vi "PI_GCS3_Sample_Application_Motion.vi"() -> ()   [LabVIEW 2020]
doc: "This VI demonstrates how to initialize a PI GCS3 system and how to query the help answer. \nThe diagram shows how to combine the driver VIs for these tasks. \n\nWarning: Before running this VI, modify the interface settings on the block diagram to reflect your configuration. The predefined settings provided with the VI probably do not match your system.\n\nCompatibility: This sample requires a PI GCS 3.0 controller."
uses:
  Interface Settings.ctl
  ModeOfOperation.ctl
panel:
  out "All axes on target?":bool
  out "All axes referenced?":bool
  out "Axes available?":bool caption="Any axes available?"
  out "Axis on target?":bool[](array[boolean])
  out "Referenced?":bool[](array[boolean])
  out "Any axes moving?":bool
  in  "Target Position":dbl[](array[numeric]) format="%.6f"
  out "Current Position":dbl[](array[numeric]) format="%.6f"
  in  "stop":bool
  in  "error in":errorcluster
  out "Running":bool caption="Configuration_Setup.vi is running"
  out "error out":errorcluster
  out "Conn. Axis":string[](array[string])
  out "Identification":string
  # "This VI demonstrates how to initialize a PI GCS3 system and how to move your axes.\nThe diagram shows how to combine the driver VIs for these tasks. \n\nWarning: Before running this VI, modify the interface settings on the block diagram to reflect your configuration.\n                 The predefined settings provided with the VI probably do not match your system.\n\nCompatibility: This sample requires a PI GCS 3.0 controller."
  # "Set the number of target positions\naccording to your connected axes."
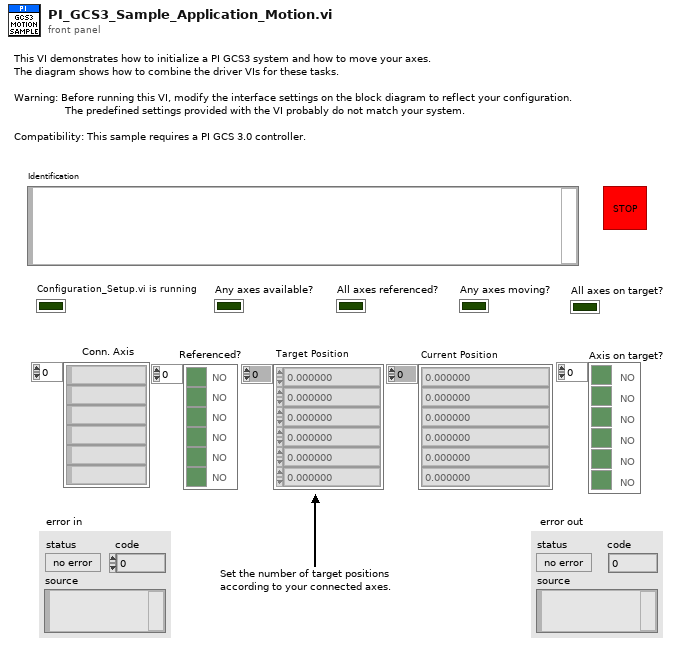
[diagram p1: front panel]
types:
  T1 = typedef "ModeOfOperation.ctl" = enum16{"Open", "Open-Loop Position", "Closed-Loop Position", "Open-Loop Velocity", "Closed-Loop Velocity", "Open-Loop Force", "Closed-Loop Force", "Step Operation"}
  T2 = typedef "Interface Settings.ctl" = cluster{"Interface":u16, "Timeout":u32, "RS232 settings":cluster{"Portnumber":u8, "Baudrate":u16}, "TCP/IP settings":cluster{"Host address/name":string, "Port":i32, "Board":i32, "TCP/IP Search?":bool}, "USB settings":cluster{"S/N":string, "USB Search?":bool}, "DaisyChain settings":cluster{"Register DC":bool, "DaisyChain Search?":bool, "Device ID":i32}, "DLL for Device":u16}
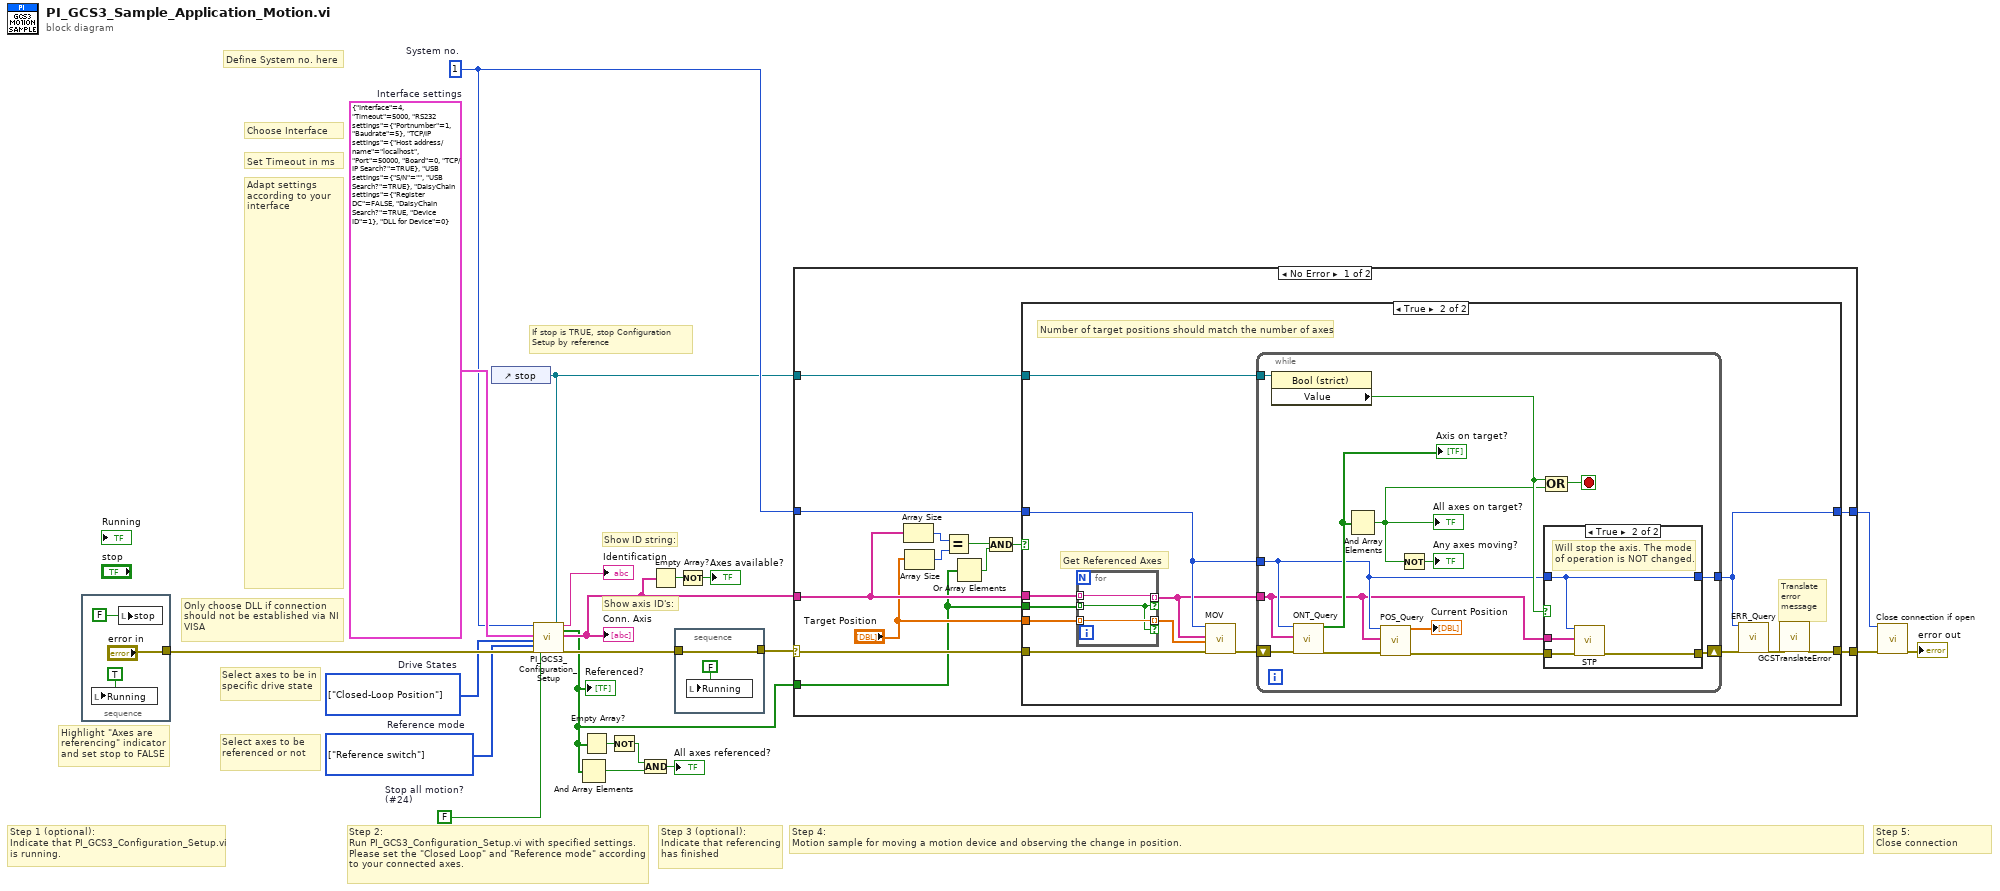
[diagram p0: block diagram]
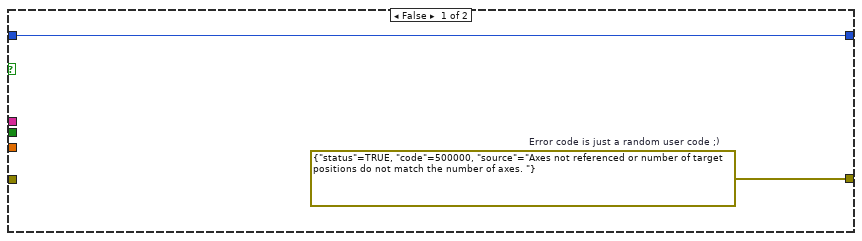
[diagram p2: hidden frame]
diagram:
  w1 = enum16{"Do not reference", "Reference switch"}[] [enum."Reference switch"] items=["Do not reference", "Reference switch"]  # Reference mode
  w2 = T1[] [enum."Closed-Loop Position"] items=["Open", "Open-Loop Position", "Closed-Loop Position", "Open-Loop Velocity", "Closed-Loop Velocity", "Open-Loop Force", "Closed-Loop Force", "Step Operation"]  # Drive States
  w16 = T2 {"Interface"=4, "Timeout"=5000, "RS232 settings"={"Portnumber"=1, "Baudrate"=5}, "TCP/IP settings"={"Host address/name"="localhost", "Port"=50000, "Board"=0, "TCP/IP Search?"=TRUE}, "USB settings"={"S/N"="", "USB Search?"=TRUE}, "DaisyChain settings"={"Register DC"=FALSE, "DaisyChain Search?"=TRUE, "Device ID"=1}, "DLL for Device"=0}  # Interface settings
  w17 = FALSE  # Stop all motion? (#24)
  w13 = 1  # System no.
  # "Step 5:\nClose connection"
  # "Define System no. here"
  # "Select axes to be referenced or not"
  # "Select axes to be in specific drive state"
  # "Adapt settings according to your interface"
  # "Set Timeout in ms"
  # "Choose Interface"
  # "Only choose DLL if connection should not be established via NI VISA"
  # "If stop is TRUE, stop Configuration\nSetup by reference"
  # "Step 4: \nMotion sample for moving a motion device and observing the change in position."
  # "Step 3 (optional): \nIndicate that referencing has finished"
  # "Step 2: \nRun PI_GCS3_Configuration_Setup.vi with specified settings.\nPlease set the \"Closed Loop\" and \"Reference mode\" according\nto your connected axes."
  # "Step 1 (optional): \nIndicate that PI_GCS3_Configuration_Setup.vi is running."
  # "Highlight \"Axes are\nreferencing\" indicator\nand set stop to FALSE"
  # "Show axis ID's:"
  # "Show ID string:"
  n1 = stacked-sequence {
    tunnel: ["error in"] -> w20
    frame #0 {
      n2 = local write "Running"(TRUE ("Running")) -> ()
      n3 = local write "stop"(FALSE ("stop")) -> ()
    }
  }
  n4 = control-ref of="stop"() -> (w12:refnum<vi>)
  n5 = call "PI_GCS3_Configuration_Setup.vi"("System no."=w13, "Interface settings"=w16, "Mode of operation"=w2, "Reference mode"=w1, "error in"=w20, "Stop all motion?"=w17, "Stop refnum"=w12) -> ("Identification"=→"Identification":string, "Referenced?"=w6:bool[], "Conn. axis"=w8:string[], "error out"=w19:errorcluster)  [unwired: 7 in, 2 out]
  "Conn. Axis" <- w8
  "Referenced?" <- w6
  n6 = And Array Elements(Boolean array=w6) -> (logical AND=w3:bool)
  n7 = Empty Array?(array=w6) -> (empty?=w7:bool)
  n8 = Not(x=w7) -> (.not. x?=w4:bool)
  n9 = And(x=w4, y=w3) -> (x .and. y?=→"All axes referenced?":bool)
  n10 = Empty Array?(array=w8) -> (empty?=w10:bool)
  n11 = stacked-sequence {
    tunnel: w19 -> [w25]
    tunnel: [w25] -> w15
    frame #0 {
      n12 = local write "Running"(FALSE ("Running")) -> ()
    }
  }
  n13 = Not(x=w10) -> (.not. x?=→"Axes available?":bool)
  n14 = case shown="No Error" w15 {
    selector: w15 -> [w28 w79]
    tunnel: [w39 w79] -> w11
    tunnel: w13 -> [w37 w78]
    tunnel: [w38 w78] -> w14
    tunnel: w8 -> [w35 _]
    tunnel: w12 -> [w36 _]
    tunnel: w6 -> [w27 _]
    frame No Error {
      n15 = Array Size(array=w35) -> (size(s)=w33:i32)
      n16 = Array Size(array="Target Position") -> (size(s)=w32:i32)
      n17 = Equal?(x=w33, y=w32) -> (x = y?=w31:bool)
      n18 = Or Array Elements(Boolean array=w27) -> (logical OR=w29:bool)
      n19 = And(x=w31, y=w29) -> (x .and. y?=w30:bool)
      n20 = case shown="True" w30 {
        tunnel: [w40 w54] -> w39
        tunnel: w28 -> [_ w52]
        tunnel: [w41 w50] -> w38
        tunnel: w35 -> [_ w49]
        tunnel: w27 -> [_ w48]
        tunnel: w37 -> [w41 w47]
        tunnel: w36 -> [_ w45]
        tunnel: "Target Position" -> [_ w43]
        frame False {
          w40 = errorcluster {"status"=TRUE, "code"=500000, "source"="Axes not referenced or number of target positions do not match the number of axes. "}  # Error code is just a random user code ;)
        }
        frame True {
          # "Number of target positions should match the number of axes"
          # "Get Referenced Axes"
          # "Translate\nerror \nmessage"
          n21 = for {
            tunnel: w49 -> [w57] mode=indexing
            tunnel: w48 -> [w55] mode=indexing
            tunnel: [w57] -> w46 mode=indexing if=w55
            tunnel: [w56] -> w42 mode=indexing if=w55
            tunnel: w43 -> [w56] mode=indexing
          }
          n22 = call "MOV.vi"("System no."=w47, "Axes to move"=w46, "Position values"=w42, "error in"=w52) -> ("error out"=w44:errorcluster)  [unwired: 1 in, 14 out]
          n23 = while {
            shift-right: [w69] -> w51
            shift-left: w44 -> [w63]
            tunnel: w45 -> [w68]
            tunnel: w47 -> [w62]
            tunnel: w46 -> [w61]
            tunnel: [w64] -> w50
            stop <- w67 stop-if-true
            n24 = property class="Bool (strict)"(reference=w68) -> ("Value"=w66:bool)  [unwired: 1 in, 2 out]
            n25 = call "ONT_Query.vi"("System no."=w62, "Axes to query"=w61, "error in"=w63) -> ("Axis on target?"=w65:bool[], "error out"=w71:errorcluster)  [unwired: 2 in, 13 out]
            "Axis on target?" <- w65
            n26 = And Array Elements(Boolean array=w65) -> (logical AND=w58:bool)
            "All axes on target?" <- w58
            n27 = call "POS_Query.vi"("System no."=w62, "Axes to query"=w61, "error in"=w71) -> ("Position"=→"Current Position":dbl[], "error out"=w70:errorcluster)  [unwired: 2 in, 13 out]
            n28 = Not(x=w58) -> (.not. x?=→"Any axes moving?":bool)
            n29 = case shown="True" w66 {
              tunnel: w70 -> [w73 w76]
              tunnel: [w73 w75] -> w69
              tunnel: w62 -> [w72 w77]
              tunnel: [w72 w77] -> w64
              tunnel: w61 -> [_ w74]
              frame False {
              }
              frame True {
                # "Will stop the axis. The mode of operation is NOT changed."
                n30 = call "STP.vi"("System no."=w77, "Affected axes?"=w74, "error in"=w76) -> ("error out"=w75:errorcluster)  [unwired: 16 in]
              }
            }
            n31 = Compound Arithmetic op=OR(w66, w58) -> (w67:bool)
          }
          n32 = call "ERR_Query.vi"("System no."=w50, "error in"=w51) -> ("error out"=w53:errorcluster)  [unwired: 17 out]
          n33 = call "GCSTranslateError.vi"("error in"=w53) -> ("error out"=w54:errorcluster)  [unwired: 18 out]
        }
      }
    }
    frame Error {
      # "Error during initialization"
    }
  }
  n34 = call "Close connection if open.vi"("System no."=w14, "error in"=w11) -> ("error out"=→"error out":errorcluster)  [unwired: 1 in, 16 out]
